vi "Match_Spec.vi"(8 "error in (no error)":errorcluster caption="에러 입력(에러 없음)", 10 "DATA IN":string[][](array[string]), 11 "SPEC IN":string[][](array[string])) -> (0 "error out":errorcluster caption="에러 출력", 2 "에러?":bool, 3 "Spec Out":string[][](array[string]))   [LabVIEW 2020]
panel:
  # "0 : FUNC\n1 : FUNC_EXT\n2 : FUNC_CON\n3 : C1_LOW\n4 : C1_LUNIT\n5 : C1_LCON\n6 : C1_HIGH\n7 : C1_HUNIT\n8 : C1_HCON\n9 : RANGE_LOW\n10 : RANGE_LUNIT\n11 : RANGE_LDIV\n12 : RANGE_HIGH\n13 : RANGE_HUNIT\n14 : RANGE_HDIV\n15 : SPEC_VAL\n16 : SPEC_VAL\n17 : SPEC_UNIT"
  # "0 : FUNC\n1 : FUNC_EXT\n2 : FUNC_CON\n3 : C1_VAL\n4 : C1_UNIT\n5 : RANGE_VAL\n6 : RANGE_UNIT"
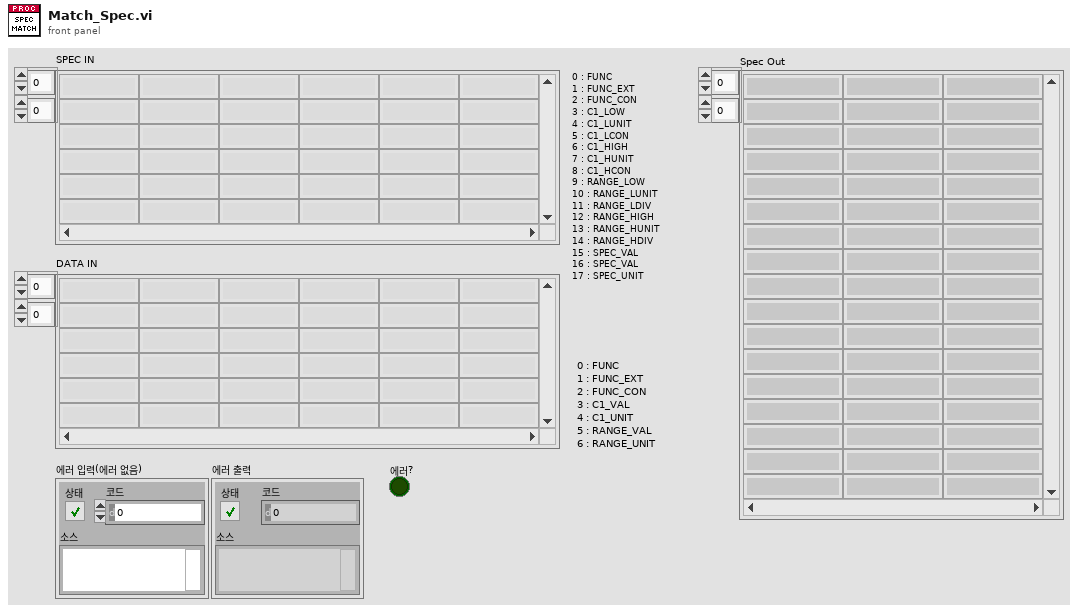
[diagram p1: front panel]
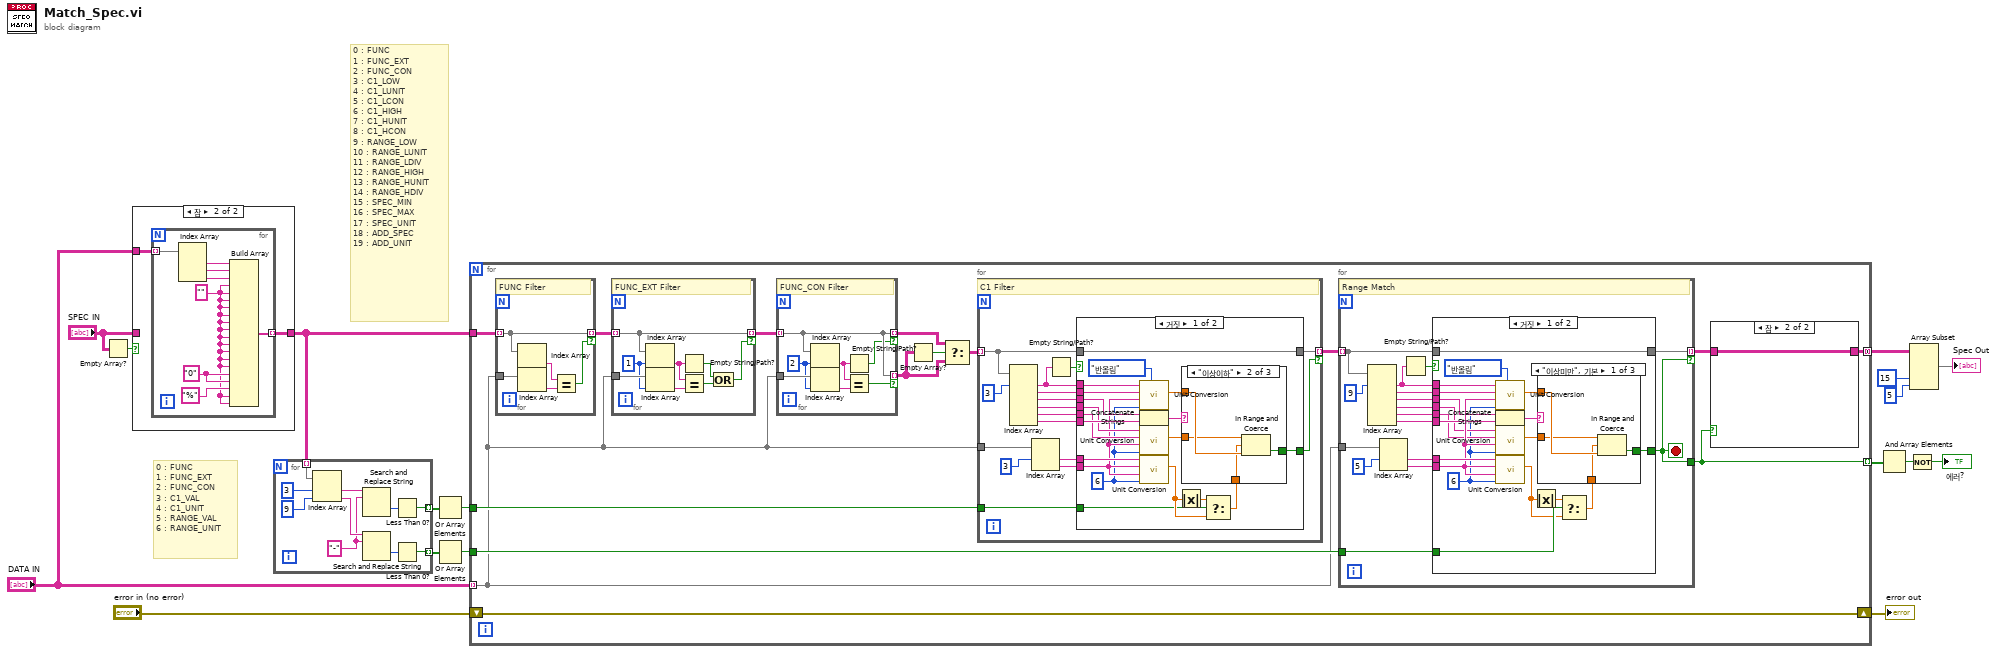
[diagram p0: block diagram]
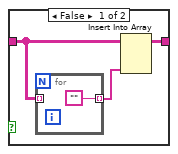
[diagram p3: hidden frame]
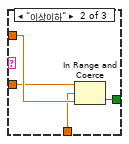
[diagram p4: hidden frame]
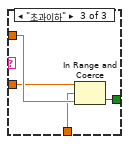
[diagram p5: hidden frame]
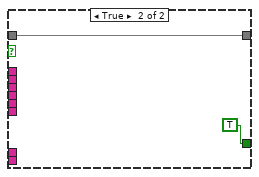
[diagram p6: hidden frame]
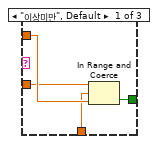
[diagram p7: hidden frame]
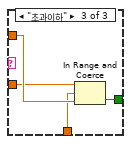
[diagram p8: hidden frame]
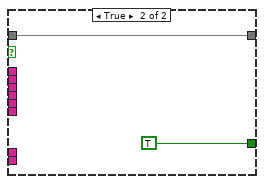
[diagram p9: hidden frame]
diagram:
  # "0 : FUNC\n1 : FUNC_EXT\n2 : FUNC_CON\n3 : C1_VAL\n4 : C1_UNIT\n5 : RANGE_VAL\n6 : RANGE_UNIT"
  # "0 : FUNC\n1 : FUNC_EXT\n2 : FUNC_CON\n3 : C1_LOW\n4 : C1_LUNIT\n5 : C1_LCON\n6 : C1_HIGH\n7 : C1_HUNIT\n8 : C1_HCON\n9 : RANGE_LOW\n10 : RANGE_LUNIT\n11 : RANGE_LDIV\n12 : RANGE_HIGH\n13 : RANGE_HUNIT\n14 : RANGE_HDIV\n15 : SPEC_MIN\n16 : SPEC_MAX\n17 : SPEC_UNIT\n18 : ADD_SPEC\n19 : ADD_UNIT"
  n1 = Empty Array?(array="SPEC IN") -> (empty?=w4:bool)
  n2 = case shown="참" w4 {
    tunnel: "SPEC IN" -> [w18 _]
    tunnel: [w18 w19] -> w2
    tunnel: "DATA IN" -> [_ w20]
    frame False {
    }
    frame True {
      n3 = for {
        tunnel: w20 -> [w28] mode=indexing
        tunnel: [w21] -> w19 mode=indexing
        w23 = "0" ("원소")
        w22 = "" ("원소")
        n4 = Index Array(array=w28) -> (element #1=w27:string, element #2=w26:string, element #3=w25:string)  [unwired: 3 in]
        n5 = Build Array(w27, w26, w25, w22, w22, w22, w22, w22, w22, w22, w22, w22, w22, w22, w22, w23, w23, "%" ("원소"), w22, w22) -> (w21:string[])
      }
    }
  }
  n6 = for {
    tunnel: w2 -> [w38] mode=indexing
    tunnel: [w34] -> w8 mode=indexing
    tunnel: [w29] -> w6 mode=indexing
    w31 = "-" ("검색 문자열")
    n7 = Index Array(array=w38, index #1=3 ("비활성화된 인덱스 (열)"), index #2=9 ("비활성화된 인덱스 (열)")) -> (element #1=w32:string, element #2=w36:string)
    n8 = Search and Replace String(input string=w32, search string=w31) -> (offset past replacement=w30:i32)  [unwired: 6 in, 3 out]
    n9 = Search and Replace String(input string=w36, search string=w31) -> (offset past replacement=w35:i32)  [unwired: 6 in, 3 out]
    n10 = Less Than 0?(x=w30) -> (x < 0?=w29:bool)
    n11 = Less Than 0?(x=w35) -> (x < 0?=w34:bool)
  }
  n12 = Or Array Elements(Boolean array=w6) -> (logical OR=w5:bool)
  n13 = Or Array Elements(Boolean array=w8) -> (logical OR=w7:bool)
  n14 = for {
    tunnel: "DATA IN" -> [w44] mode=indexing
    tunnel: w2 -> [w53]
    tunnel: [w47] -> w12 mode=concatenating
    shift-right: [w50] -> w16
    shift-left: "error in (no error)" -> [w50]
    tunnel: [w49] -> w15 mode=indexing
    tunnel: w7 -> [w46]
    tunnel: w5 -> [w45]
    n15 = for {
      tunnel: w53 -> [w175] mode=indexing
      tunnel: w44 -> [w176]
      tunnel: [w175] -> w52 mode=indexing if=w174
      # "FUNC Filter"
      n16 = Index Array(array=w175) -> (element=w173:string)  [unwired: 1 in]
      n17 = Index Array(array=w176) -> (element=w172:string)  [unwired: 1 in]
      n18 = Equal?(x=w173, y=w172) -> (x = y?=w174:bool)
    }
    n19 = for {
      tunnel: w52 -> [w170] mode=indexing
      tunnel: w44 -> [w171]
      tunnel: [w170] -> w43 mode=indexing if=w166
      w164 = 1 ("인덱스")
      # "FUNC_EXT Filter"
      n20 = Index Array(array=w170, index=w164) -> (element=w167:string)
      n21 = Index Array(array=w171, index=w164) -> (element=w168:string)
      n22 = Empty String/Path?(string/path=w167) -> (empty?=w165:bool)
      n23 = Equal?(x=w167, y=w168) -> (x = y?=w169:bool)
      n24 = Or(x=w165, y=w169) -> (x .or. y?=w166:bool)
    }
    n25 = for {
      tunnel: w44 -> [w60]
      tunnel: [w56] -> w41 mode=indexing if=w54
      tunnel: w43 -> [w56] mode=indexing
      tunnel: [w56] -> w39 mode=indexing if=w55
      w57 = 2 ("인덱스")
      # "FUNC_CON Filter"
      n26 = Index Array(array=w56, index=w57) -> (element=w58:string)
      n27 = Index Array(array=w60, index=w57) -> (element=w59:string)
      n28 = Empty String/Path?(string/path=w58) -> (empty?=w54:bool)
      n29 = Equal?(x=w58, y=w59) -> (x = y?=w55:bool)
    }
    n30 = Empty Array?(array=w39) -> (empty?=w42:bool)
    n31 = Select(t=w41, s=w42, f=w39) -> (s? t:f=w40:string[][])
    n32 = for {
      tunnel: w40 -> [w127] mode=indexing
      tunnel: w44 -> [w130]
      tunnel: [w126] -> w51 mode=indexing if=w120
      tunnel: w45 -> [w115]
      # "C1 Filter"
      n33 = Index Array(array=w127, index #1=3 ("인덱스")) -> (element #1=w124:string, element #2=w123:string, element #3=w121:string, element #4=w118:string, element #5=w117:string, element #6=w119:string)  [unwired: 5 in]
      n34 = Index Array(array=w130, index #1=3 ("인덱스")) -> (element #1=w125:string, element #2=w122:string)  [unwired: 1 in]
      n35 = Empty String/Path?(string/path=w124) -> (empty?=w128:bool)
      n36 = case shown="거짓" w128 {
        tunnel: w127 -> [w136 w163]
        tunnel: [w136 w163] -> w126
        tunnel: w125 -> [w140 _]
        tunnel: w124 -> [w149 _]
        tunnel: w123 -> [w148 _]
        tunnel: w122 -> [w139 _]
        tunnel: w121 -> [w147 _]
        tunnel: [w138 TRUE] -> w120
        tunnel: w119 -> [w146 _]
        tunnel: w118 -> [w143 _]
        tunnel: w117 -> [w142 _]
        tunnel: w115 -> [w131 _]
        frame False {
          w137 = i8 6 ("소수점 자리수")
          w135 = enum16{"없음", "반올림", "올림", "내림"}."반올림" ("반올림 옵션")
          n37 = call "Unit Conversion.vi"("반올림 옵션"=w135, "소수점 자리수"=w137, "환산단위"=w139, "입력단위"=w148, "입력값"=w149) -> ("환산값 (DBL)"=w144:dbl)  [unwired: 1 in, 5 out]
          n38 = Concatenate Strings(w147, w146) -> (w145:string)
          n39 = call "Unit Conversion.vi"("반올림 옵션"=w135, "소수점 자리수"=w137, "환산단위"=w139, "입력단위"=w142, "입력값"=w143) -> ("환산값 (DBL)"=w141:dbl)  [unwired: 1 in, 5 out]
          n40 = call "Unit Conversion.vi"("반올림 옵션"=w135, "소수점 자리수"=w137, "환산단위"=w139, "입력단위"=w139, "입력값"=w140) -> ("환산값 (DBL)"=w133:dbl)  [unwired: 1 in, 5 out]
          n41 = Absolute Value(x=w133) -> (abs(x)=w134:dbl)
          n42 = Select(t=w134, s=w131, f=w133) -> (s? t:f=w132:dbl)
          n43 = case shown="\"이상이하\"" w145 {
            tunnel: w144 -> [w153 w156 w161]
            tunnel: w141 -> [w152 w155 w159]
            tunnel: w132 -> [w151 w154 w160]
            tunnel: [w150 w157 w158] -> w138
            frame "이상미만", Default {
              n44 = In Range and Coerce(upper limit=w152, x=w151, lower limit=w153) -> (In Range?=w150:bool)  [unwired: 1 out]
            }
            frame "이상이하" {
              n45 = In Range and Coerce(upper limit=w155, x=w154, lower limit=w156) -> (In Range?=w157:bool)  [unwired: 1 out]
            }
            frame "초과이하" {
              n46 = In Range and Coerce(upper limit=w159, x=w160, lower limit=w161) -> (In Range?=w158:bool)  [unwired: 1 out]
            }
          }
        }
        frame True {
        }
      }
    }
    n47 = for {
      tunnel: w51 -> [w70] mode=indexing
      tunnel: w44 -> [w81]
      tunnel: [w69] -> w48 mode=indexing if=w71
      tunnel: [w71] -> w49
      tunnel: w46 -> [w66]
      stop <- w71 stop-if-true
      # "Range Match"
      n48 = Index Array(array=w70, index #1=9 ("인덱스")) -> (element #1=w68:string, element #2=w78:string, element #3=w76:string, element #4=w74:string, element #5=w73:string, element #6=w75:string)  [unwired: 5 in]
      n49 = Index Array(array=w81, index #1=5 ("인덱스")) -> (element #1=w79:string, element #2=w77:string)  [unwired: 1 in]
      n50 = Empty String/Path?(string/path=w68) -> (empty?=w67:bool)
      n51 = case shown="거짓" w67 {
        tunnel: w79 -> [w100 _]
        tunnel: w68 -> [w99 _]
        tunnel: w78 -> [w98 _]
        tunnel: w77 -> [w97 _]
        tunnel: w76 -> [w96 _]
        tunnel: w75 -> [w95 _]
        tunnel: w74 -> [w94 _]
        tunnel: w73 -> [w93 _]
        tunnel: [w87 TRUE] -> w71
        tunnel: w70 -> [w86 w114]
        tunnel: [w86 w114] -> w69
        tunnel: w66 -> [w85 _]
        frame False {
          w88 = i8 6 ("소수점 자리수")
          w89 = enum16{"없음", "반올림", "올림", "내림"}."반올림" ("반올림 옵션")
          n52 = call "Unit Conversion.vi"("반올림 옵션"=w89, "소수점 자리수"=w88, "환산단위"=w97, "입력단위"=w98, "입력값"=w99) -> ("환산값 (DBL)"=w91:dbl)  [unwired: 1 in, 5 out]
          n53 = Concatenate Strings(w96, w95) -> (w92:string)
          n54 = call "Unit Conversion.vi"("반올림 옵션"=w89, "소수점 자리수"=w88, "환산단위"=w97, "입력단위"=w93, "입력값"=w94) -> ("환산값 (DBL)"=w90:dbl)  [unwired: 1 in, 5 out]
          n55 = call "Unit Conversion.vi"("반올림 옵션"=w89, "소수점 자리수"=w88, "환산단위"=w97, "입력단위"=w97, "입력값"=w100) -> ("환산값 (DBL)"=w84:dbl)  [unwired: 1 in, 5 out]
          n56 = Absolute Value(x=w84) -> (abs(x)=w83:dbl)
          n57 = Select(t=w83, s=w85, f=w84) -> (s? t:f=w82:dbl)
          n58 = case shown="\"이상미만\", 기본" w92 {
            tunnel: w91 -> [w104 w107 w112]
            tunnel: w90 -> [w103 w106 w110]
            tunnel: w82 -> [w102 w105 w111]
            tunnel: [w101 w108 w109] -> w87
            frame "이상미만", Default {
              n59 = In Range and Coerce(upper limit=w103, x=w102, lower limit=w104) -> (In Range?=w101:bool)  [unwired: 1 out]
            }
            frame "이상이하" {
              n60 = In Range and Coerce(upper limit=w106, x=w105, lower limit=w107) -> (In Range?=w108:bool)  [unwired: 1 out]
            }
            frame "초과이하" {
              n61 = In Range and Coerce(upper limit=w110, x=w111, lower limit=w112) -> (In Range?=w109:bool)  [unwired: 1 out]
            }
          }
        }
        frame True {
        }
      }
    }
    n62 = case shown="참" w49 {
      tunnel: w48 -> [w63 w65]
      tunnel: [w62 w65] -> w47
      frame False {
        n63 = for {
          tunnel: [""] -> w61 mode=indexing
          tunnel: w63 -> [_] mode=indexing
        }
        n64 = Insert Into Array(array=w63, new element=w61) -> (w62:string[][])  [unwired: 2 in]
      }
      frame True {
      }
    }
  }
  "error out" <- w16
  n65 = And Array Elements(Boolean array=w15) -> (logical AND=w14:bool)
  n66 = Not(x=w14) -> (.not. x?=→"에러?":bool)
  n67 = Array Subset(array=w12, index (col)=15 ("인덱스"), length (col)=5 ("길이")) -> (→"Spec Out":string[][])  [unwired: 2 in]
